vi "Basic Set Regulation.vi"() -> ()   [LabVIEW 2016]
doc: "Purpose: This example shows how to set a sensor regulation and generate a sinusoidal profile on the first sensor and pressure module of the chain\nHardware setup: At least one Fluigent pressure controller (MFCS, MFCS-EZ or FlowEZ) and at least one Fluigent sensor (flow-unit connected to FRP or FlowEZ)"
uses:
  fgt_SDK.lvlib
  <vilib>/ptbypt/NI_PtbyPt.lvlib
panel:
  out "Waveform Chart":cluster{"sine wave":dbl, "value out":sgl}(graph)
  in  "Boolean":bool
  out "error out":errorcluster
  # "Hit the \"Run\" button to start generating a flow sinewave"
  # "Hit the \"Run\" button to start the regulation"
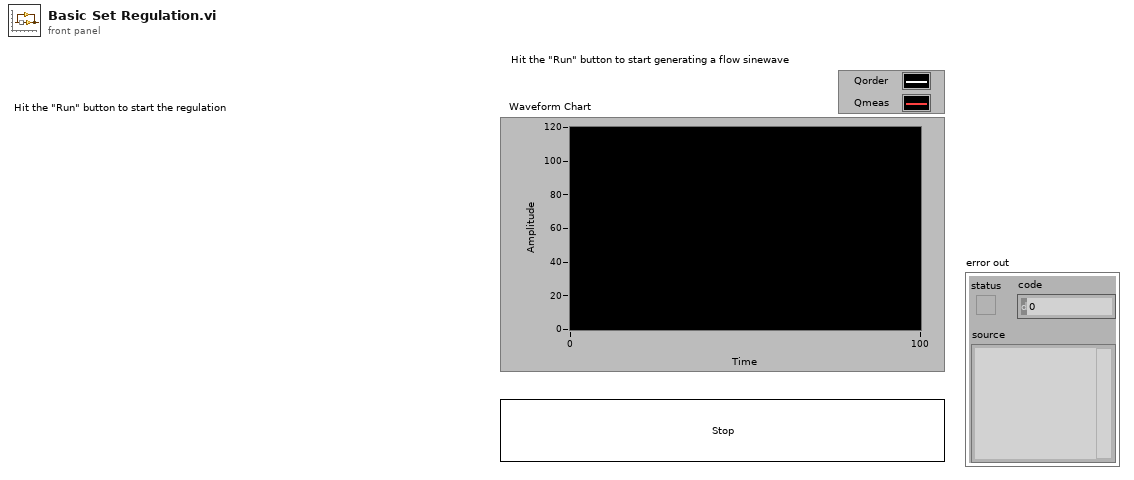
[diagram p1: front panel]
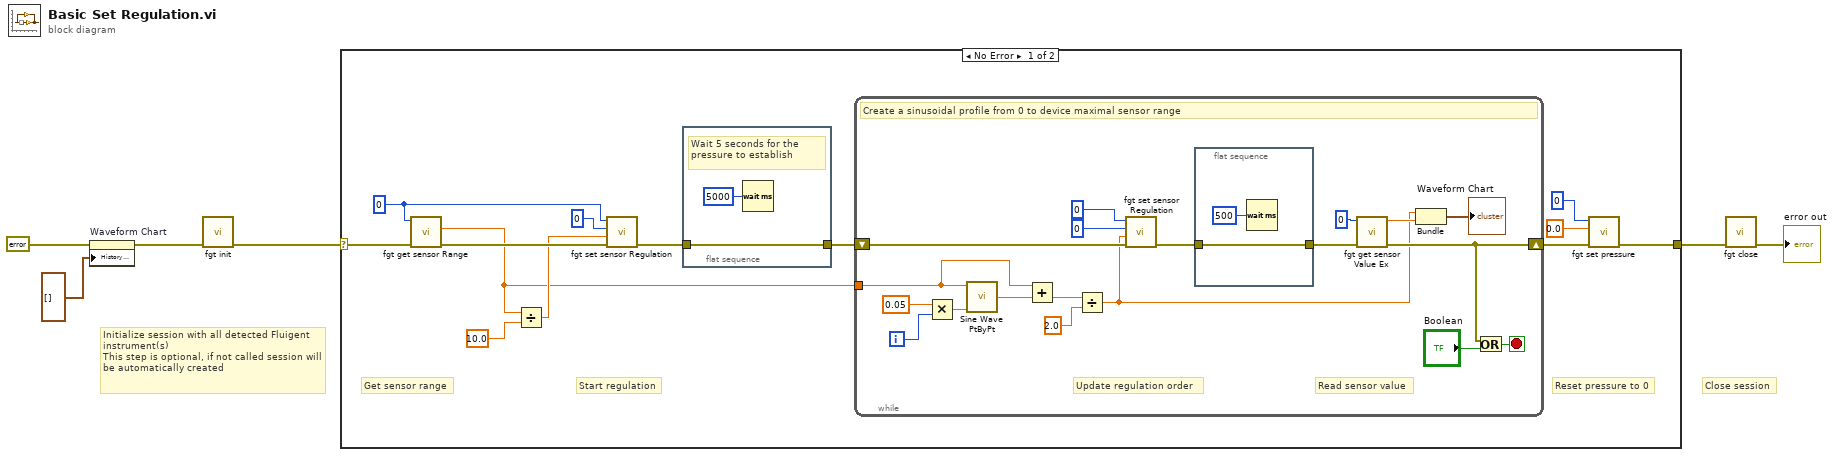
[diagram p0: block diagram]
diagram:
  # "Close session"
  # "Initialize session with all detected Fluigent instrument(s)\nThis step is optional, if not called session will be automatically created"
  n1 = property on="Waveform Chart" class="WFChart (strict)"(error in=errorcluster {"status"=FALSE, "code"=0, "source"=""} ("error in (no error)"), "History Data"=cluster{"sine wave":dbl, "value out":sgl}[] []) -> (error out=w2:errorcluster)  [unwired: 1 in, 1 out]
  n2 = call "fgt init.vi"("error in (no error)"=w2) -> ("error out"=w6:errorcluster)  [unwired: 10 in]
  n3 = case shown="No Error" w6 {
    selector: w6 -> [w16 w43]
    tunnel: [w17 w43] -> w5
    frame No Error {
      w14 = u32 0 ("sensorIndex")
      # "Start regulation"
      # "Get sensor range"
      # "Reset pressure to 0"
      n4 = call "fgt get sensor Range.vi"("error in (no error)"=w16, "sensorIndex"=w14) -> ("error out"=w15:errorcluster, "Smax out"=w9:sgl)  [unwired: 7 in, 1 out]
      n5 = Divide(x=w9, y=sgl 10.0) -> (x/y=w11:sgl)
      n6 = call "fgt set sensor Regulation.vi"("error in (no error)"=w15, "setpoint"=w11, "pressureIndex"=u32 0, "sensorIndex"=w14) -> ("error out"=w10:errorcluster)  [unwired: 7 in]
      n7 = flat-sequence {
        tunnel: w10 -> [w41]
        tunnel: [w41] -> w8
        frame #0 {
          # "Wait 5 seconds for the pressure to establish"
          n8 = Wait (ms)(milliseconds to wait=u32 5000) -> ()  [unwired: 1 out]
        }
      }
      n9 = while {
        tunnel: w9 -> [w22]
        shift-right: [w24] -> w7
        shift-left: w8 -> [w34]
        i -> [w37]
        stop <- w25 stop-if-true
        # "Read sensor value"
        # "Update regulation order"
        # "Create a sinusoidal profile from 0 to device maximal sensor range"
        n10 = Multiply(x=0.05 ("time"), y=w37) -> (x*y=w36:dbl)
        n11 = call <vilib>:"Sine Wave PtByPt.vi"("time"=w36, "amplitude"=w22) -> ("sine wave"=w28:dbl)  [unwired: 2 in]
        n12 = Add(x=w22, y=w28) -> (x+y=w23:dbl)
        n13 = Divide(x=w23, y=2.0) -> (x/y=w21:dbl)
        n14 = call "fgt set sensor Regulation.vi"("error in (no error)"=w34, "setpoint"=w21, "pressureIndex"=u32 0, "sensorIndex"=u32 0) -> ("error out"=w31:errorcluster)  [unwired: 7 in]
        n15 = flat-sequence {
          tunnel: [w39] -> w30
          tunnel: w31 -> [w39]
          frame #0 {
            n16 = Wait (ms)(milliseconds to wait=u32 500 ("attente (ms)")) -> ()  [unwired: 1 out]
          }
        }
        n17 = call "fgt get sensor Value Ex.vi"("error in (no error)"=w30, "sensorIndex"=u32 0) -> ("error out"=w24:errorcluster, "value out"=w27:sgl)  [unwired: 7 in, 1 out]
        n18 = Bundle(w21, "value out"=w27) -> (→"Waveform Chart":cluster{dbl, "value out":sgl})  [unwired: 1 in]
        n19 = Or(x=w24, y="Boolean") -> (x .or. y?=w25:bool)
      }
      n20 = call "fgt set pressure.vi"("error in (no error)"=w7, "pressure"=sgl 0.0, "pressureIndex"=u32 0) -> ("error out"=w17:errorcluster)  [unwired: 8 in]
    }
    frame Error {
    }
  }
  n21 = call "fgt close.vi"("error in (no error)"=w5) -> ("error out"=→"error out":errorcluster)  [unwired: 10 in]
